vi "getQueue.vi"(2 "queue msg":string, 3 "ROS in":T1) -> (1 "ROS out":T1)   [LabVIEW 2010]
doc: "Attempts to obtain a reference to the queue at name until 5 seconds has passed, when it times out."
uses:
  <userlib>/ROSforLV_0.1/ROS/Code/SubVIs/_ROSControl.ctl
  <userlib>/ROSforLV_0.1/ROS/Code/SubVIs/_ROSDirection.ctl
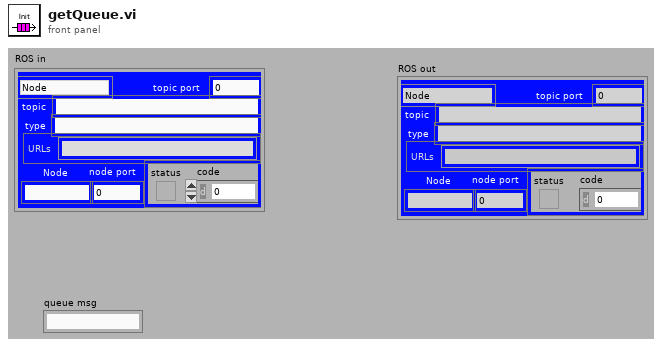
[diagram p1: front panel]
types:
  T1 = typedef "_ROSControl.ctl" = cluster{"topic port":u16, "Node":string, "topic":string, "type":string, "node port":u32, "error ":errorcluster, "Direction":T2, "APIs":string[]}
  T2 = typedef "_ROSDirection.ctl" = enum16{"Node", "Publisher", "Subscriber", "Service Client"}
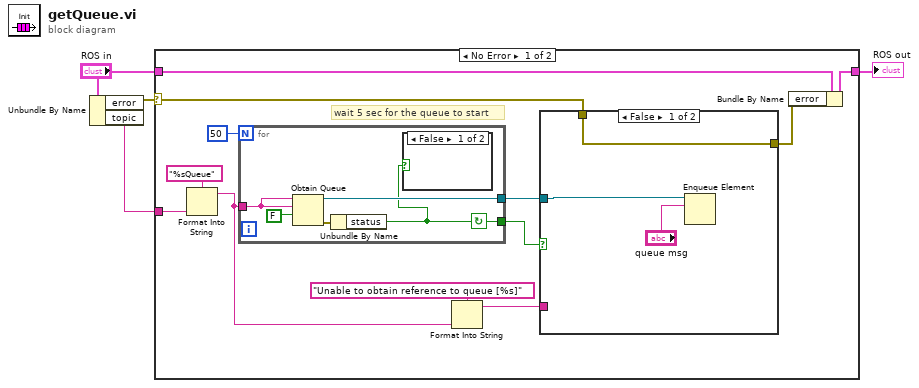
[diagram p0: block diagram]
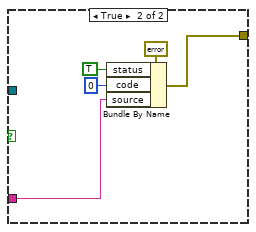
[diagram p2: hidden frame]
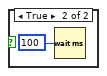
[diagram p3: hidden frame]
diagram:
  n1 = Unbundle By Name("ROS in") -> ("error"=w4:errorcluster, "topic"=w1:string)
  n2 = case shown="No Error" w4 {
    selector: w4 -> [w8 _]
    tunnel: "ROS in" -> [w11 w31]
    tunnel: [w10 w31] -> w2
    tunnel: w1 -> [w5 _]
    frame No Error {
      # "wait 5 sec for the queue to start"
      n3 = Format Into String(format string="%sQueue" ("name (unnamed)"), w5) -> (resulting string=w6:string)  [unwired: 2 in, 1 out]
      n4 = for {
        N: 50 -> [_]
        tunnel: w6 -> [w29]
        tunnel: [w27] -> w12
        tunnel: [w25] -> w15
        stop <- w25 continue-if-true
        n5 = Obtain Queue(name (unnamed)=w29, element data type=w29, create if not found? (T)=FALSE) -> (queue out=w27:refnum<queue>, error out=w26:errorcluster)  [unwired: 2 in, 1 out]
        n6 = Unbundle By Name(w26) -> ("status"=w25:bool)
        n7 = case shown="False" w25 {
          frame False {
          }
          frame True {
            n8 = Wait (ms)(milliseconds to wait=u32 100) -> ()  [unwired: 1 out]
          }
        }
      }
      n9 = Format Into String(format string="Unable to obtain reference to queue [%s]" ("source"), w6) -> (resulting string=w13:string)  [unwired: 2 in, 1 out]
      n10 = case shown="False" w15 {
        tunnel: [w18 w24] -> w9
        tunnel: w13 -> [_ w20]
        tunnel: w12 -> [w19 _]
        tunnel: w8 -> [w18 _]
        frame False {
          n11 = Enqueue Element(queue=w19, element="queue msg") -> ()  [unwired: 2 in, 3 out]
        }
        frame True {
          n12 = Bundle By Name(cluster=errorcluster {"status"=FALSE, "code"=0, "source"=""} ("error out"), "status"=TRUE, "code"=0, "source"=w20) -> (w24:errorcluster)
        }
      }
      n13 = Bundle By Name(cluster=w11, "error"=w9) -> (w10:T1)
    }
    frame Error {
    }
  }
  "ROS out" <- w2
